vi "RichToFlatnidaqmx_grpc_CreateCIFreqChanResponse.vi"(5 "OutputClusterType":T1, 11 "InputCluster":T2) -> (3 "OutputCluster":T1)   [LabVIEW 2021, in "NI_DAQmx_client.lvlib"]
uses:
  NI_DAQmx_client.lvlib
  nidaqmx_grpc_CreateCIFreqChanResponse_Flat.ctl
  nidaqmx_grpc_CreateCIFreqChanResponse.ctl
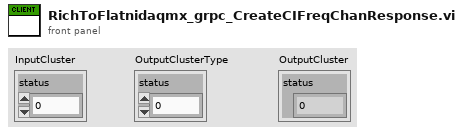
[diagram p1: front panel]
types:
  T1 = typedef "NI_DAQmx_client.lvlib/nidaqmx_grpc_CreateCIFreqChanResponse_Flat.ctl" = cluster{"status":i32}
  T2 = typedef "NI_DAQmx_client.lvlib/nidaqmx_grpc_CreateCIFreqChanResponse.ctl" = cluster{"status":i32}
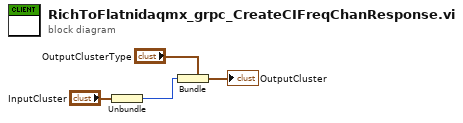
[diagram p0: block diagram]
diagram:
  n1 = Unbundle "Unbundle"("InputCluster") -> ("status"=w1:i32)
  n2 = Bundle "Bundle"(cluster="OutputClusterType", "status"=w1) -> (→"OutputCluster":T1)
